vi "PV HLT5xx Lock TF Vent.vi"(7 "Adress of unit":u16=1 min=1 max=999 step=1, 8 "error in (no error)":errorcluster, 9 "set Lock TF Vent":bool[](array[boolean])=[FALSE, FALSE, FALSE, FALSE, FALSE], 10 "Parameter\nread only<->describe":bool, 11 "VISA session":refnum<visa-resource-name>) -> (0 "error out":errorcluster, 1 "Lock TF Vent out":bool[](array[boolean]), 2 "response (data)":string, 3 "dup VISA session":refnum<visa-resource-name>)   [LabVIEW 2016, in "Pfeiffer Vacuum.lvlib"]
doc: "This VI allows you to set or check the \"Lock Twin Flow Vent (Para 663)\" on the SmartTest (HLT5xx)."
uses:
  Pfeiffer Vacuum.lvlib
panel:
  # "Lock TF Vent"
  # "Counter Flow enabled"
  # "Counter Flow enabled"
  # "Twin Flow low enabled"
  # "Twin Flow low enabled"
  # "Twin Flow high enabled"
  # "Twin Flow high enabled"
  # "Venting manuell (if Venting at Stop seated)"
  # "Venting manuell"
  # "Venting at Stop"
  # "Venting at Stop"
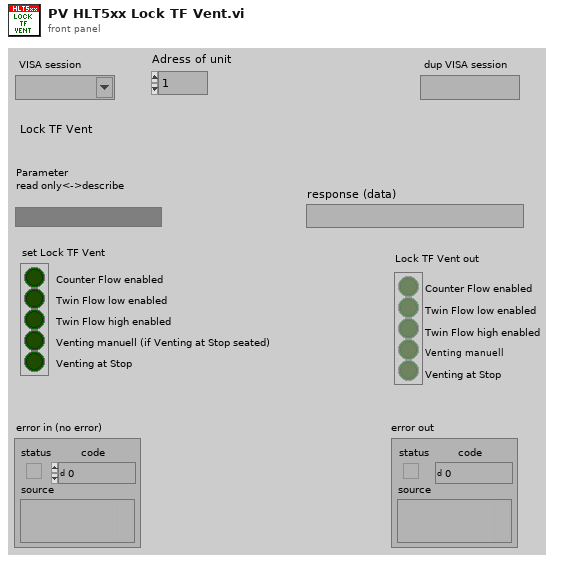
[diagram p1: front panel]
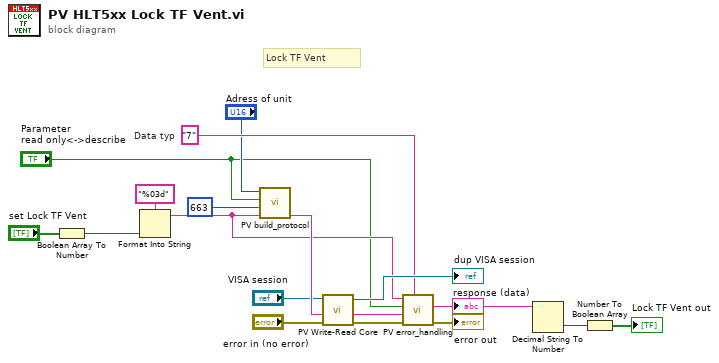
[diagram p0: block diagram]
diagram:
  w12 = "7"  # Data typ
  # "Lock TF Vent"
  n1 = Boolean Array To Number(Boolean array="set Lock TF Vent") -> (number=w1:u32)
  n2 = Format Into String(format string="%03d" ("Format-String"), w1) -> (resulting string=w13:string)  [unwired: 2 in, 1 out]
  n3 = call "PV build_protocol.vi"("Data"=w13, "Parameter-number"=u16 663, "parameter\nread<->describe"="Parameter\nread only<->describe", "Adress"="Adress of unit") -> ("output"=w17:string)  [unwired: 3 in]
  n4 = call "PV Write-Read Core.vi"("error in"="error in (no error)", "Write data in"=w17, "VISA session"="VISA session") -> ("error out"=w15:errorcluster, "response (data) out"=w16:string, "dup VISA session"=→"dup VISA session":refnum<visa-resource-name>)  [unwired: 2 in]
  n5 = call "PV error_handling.vi"("Data Typ in"=w12, "error in"=w15, "response (data) in"=w16, "Parameter\nread only<->describe"="Parameter\nread only<->describe", "data in"=w13) -> ("error out"=→"error out":errorcluster, "Data out"=w10:string)  [unwired: 4 in, 1 out]
  "response (data)" <- w10
  n6 = Decimal String To Number(string=w10) -> (number=w3:i32)  [unwired: 2 in, 1 out]
  n7 = Number To Boolean Array(number=w3) -> (Boolean array=→"Lock TF Vent out":bool[])
